vi "Drivetrain Loop.vi"(11 "Axes":T1) -> ()   [LabVIEW 2017]
uses:
  Common Code/Gamepads/Axes Cluster.ctl
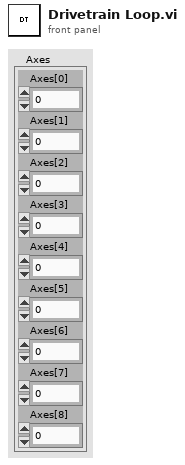
[diagram p1: front panel]
types:
  T1 = typedef "Axes Cluster.ctl" = cluster{"Axes[0]":dbl, "Axes[1]":dbl, "Axes[2]":dbl, "Axes[3]":dbl, "Axes[4]":dbl, "Axes[5]":dbl, "Axes[6]":dbl, "Axes[7]":dbl, "Axes[8]":dbl}
  T2 = typedef "WPI_MotorControlDeviceRef.ctl" = cluster{"DeviceStatus":errorcluster, "Type":T3, "PWM":cluster{"PWM Channel":T4, "DeadBand":T5}, "CAN":cluster{"Device Number":u8, "SetOutput VI Ref":variant, "GetOutput VI Ref":variant, "Enable VI Ref":variant, "Disable VI Ref":variant, "Data":variant}, "Invert":bool, "DIO PWM":cluster{"PWM \"Enable\" Channel":T4, "DIOChannel":T6, "PWM Rate":dbl}}
  T3 = typedef "WPI_MotorControlType.ctl" = enum16{"PWM", "CAN", "DIO PWM"}
  T4 = typedef "FPGA_DIOPWMChannel.ctl" = enum8{"PWM 0", "PWM 1", "PWM 2", "PWM 3", "PWM 4", "PWM 5", "PWM 6", "PWM 7", "PWM 8", "PWM 9", "PWM MXP 0", "PWM MXP 1", "PWM MXP 2", "PWM MXP 3", "PWM MXP 4", "PWM MXP 5", "PWM MXP 6", "PWM MXP 7", "PWM MXP 8", "PWM MXP 9", "Invalid"}
  T5 = typedef "WPI_PWMDeadband.ctl" = cluster{"Name":string, "maxPositivePwm":i32, "minPositivePwm":i32, "centerPwm":i32, "maxNegativePwm":i32, "minNegativePwm":i32, "angularRange":u16}
  T6 = typedef "FPGA_DIOChannel.ctl" = enum8{"DIO 0", "DIO 1", "DIO 2", "DIO 3", "DIO 4", "DIO 5", "DIO 6", "DIO 7", "DIO 8", "DIO 9", "DIO MXP 0", "DIO MXP 1", "DIO MXP 2", "DIO MXP 3", "DIO MXP 4", "DIO MXP 5", "DIO MXP 6", "DIO MXP 7", "DIO MXP 8", "DIO MXP 9", "DIO MXP 10", "DIO MXP 11", "DIO MXP 12", "DIO MXP 13", "DIO MXP 14", "DIO MXP 15", "SPI Port CS1", "SPI Port CS2", "SPI Port CS3", "SPI Port MISO", "SPI Port MOSI", "Invalid"}
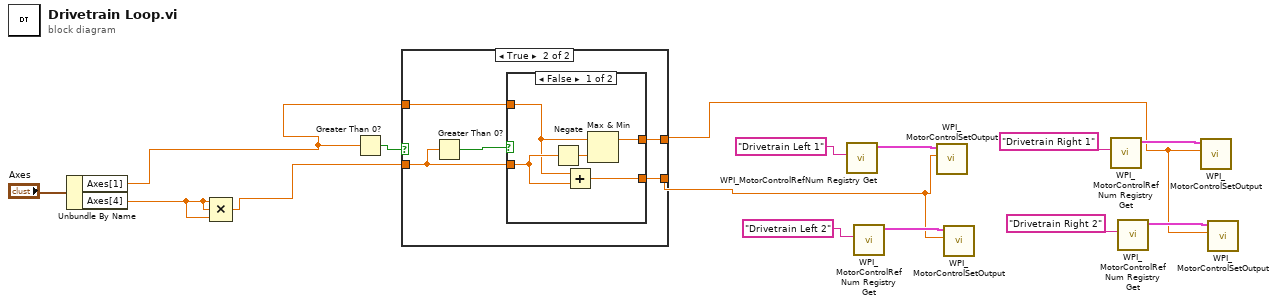
[diagram p0: block diagram]
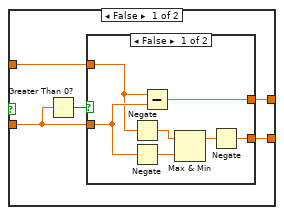
[diagram p2: hidden frame]
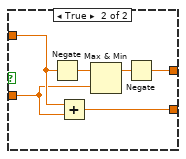
[diagram p3: hidden frame]
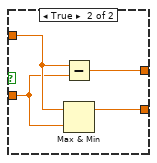
[diagram p4: hidden frame]
diagram:
  n1 = Unbundle By Name("Axes") -> ("Axes[1]"=w5:dbl, "Axes[4]"=w4:dbl)
  n2 = Compound Arithmetic op=MULTIPLY(w4, w4, w4) -> (w3:dbl)
  n3 = Greater Than 0?(x=w5) -> (x > 0?=w6:bool)
  n4 = case shown="True" w6 {
    tunnel: w3 -> [w19 w37]
    tunnel: w5 -> [w18 w36]
    tunnel: [w17 w35] -> w2
    tunnel: [w16 w34] -> w1
    frame False {
      n5 = Greater Than 0?(x=w19) -> (x > 0?=w20:bool)
      n6 = case shown="False" w20 {
        tunnel: w19 -> [w27 w29]
        tunnel: w18 -> [w25 w30]
        tunnel: [w21 w31] -> w17
        tunnel: [w22 w28] -> w16
        frame False {
          n7 = Negate(x=w25) -> (-x=w26:dbl)
          n8 = Negate(x=w27) -> (-x=w24:dbl)
          n9 = Subtract(x=w25, y=w27) -> (x-y=w21:dbl)
          n10 = Max & Min(x=w26, y=w24) -> (max(x,y)=w23:dbl)  [unwired: 1 out]
          n11 = Negate(x=w23) -> (-x=w22:dbl)
        }
        frame True {
          n12 = Negate(x=w30) -> (-x=w33:dbl)
          n13 = Add(x=w30, y=w29) -> (x+y=w28:dbl)
          n14 = Max & Min(x=w33, y=w29) -> (max(x,y)=w32:dbl)  [unwired: 1 out]
          n15 = Negate(x=w32) -> (-x=w31:dbl)
        }
      }
    }
    frame True {
      n16 = Greater Than 0?(x=w37) -> (x > 0?=w38:bool)
      n17 = case shown="False" w38 {
        tunnel: w37 -> [w43 w45]
        tunnel: w36 -> [w40 w46]
        tunnel: [w41 w44] -> w35
        tunnel: [w39 w47] -> w34
        frame False {
          n18 = Negate(x=w43) -> (-x=w42:dbl)
          n19 = Add(x=w40, y=w43) -> (x+y=w39:dbl)
          n20 = Max & Min(x=w40, y=w42) -> (max(x,y)=w41:dbl)  [unwired: 1 out]
        }
        frame True {
          n21 = Subtract(x=w46, y=w45) -> (x-y=w44:dbl)
          n22 = Max & Min(x=w46, y=w45) -> (max(x,y)=w47:dbl)  [unwired: 1 out]
        }
      }
    }
  }
  n23 = call <vilib>:"WPI_MotorControlRefNum Registry Get.vi"("refnum name"="Drivetrain Left 1") -> ("MotorControlDevRef"=w14:T2)  [unwired: 9 in, 1 out]
  n24 = call <vilib>:"WPI_MotorControlRefNum Registry Get.vi"("refnum name"="Drivetrain Left 2") -> ("MotorControlDevRef"=w11:T2)  [unwired: 9 in, 1 out]
  n25 = call <vilib>:"WPI_MotorControlSetOutput.vi"("Output"=w1, "MotorControlDevRef"=w14) -> ()  [unwired: 7 in, 3 out]
  n26 = call <vilib>:"WPI_MotorControlSetOutput.vi"("Output"=w1, "MotorControlDevRef"=w11) -> ()  [unwired: 7 in, 3 out]
  n27 = call <vilib>:"WPI_MotorControlRefNum Registry Get.vi"("refnum name"="Drivetrain Right 1") -> ("MotorControlDevRef"=w7:T2)  [unwired: 9 in, 1 out]
  n28 = call <vilib>:"WPI_MotorControlRefNum Registry Get.vi"("refnum name"="Drivetrain Right 2") -> ("MotorControlDevRef"=w10:T2)  [unwired: 9 in, 1 out]
  n29 = call <vilib>:"WPI_MotorControlSetOutput.vi"("Output"=w2, "MotorControlDevRef"=w7) -> ()  [unwired: 7 in, 3 out]
  n30 = call <vilib>:"WPI_MotorControlSetOutput.vi"("Output"=w2, "MotorControlDevRef"=w10) -> ()  [unwired: 7 in, 3 out]
